vi "LJUD_eTCValuesB.vi"(5 "aResetCounters":bool[](array[boolean]), 6 "aTimerValues Write":dbl[](array[numeric]) format="%.2f", 7 "aReadCounters":bool[](array[boolean]), 8 "error in":errorcluster, 9 "aUpdateResetTimers":bool[](array[boolean]), 10 "aReadTimers":bool[](array[boolean]), 11 "Handle In":i32) -> (0 "error out":errorcluster, 1 "aCounterValues":dbl[](array[numeric]) format="%.2f", 2 "aTimerValues Read":dbl[](array[numeric]) format="%.2f", 3 "Handle Out":i32)   [LabVIEW 2021]
doc: "This version of eTCValues uses booleans\nfor some parameters.\n\nThis is an e-function that can update\nand read all the timers and counters\nin a single call. A somewhat complex\nfunction, but can help reinforce the\ninteraction between the different timers\nand counters on the device.\n\nSee Sections 4.2 and 4.3 of the device's\ndatasheet for more information."
uses:
  labjackud.dll
panel:
  # "This version of eTCValues uses booleans\nfor some parameters.  This makes for\nmore readable programs."
  # "This version of eTCValues uses booleans\nfor some parameters.\n\nThis is an e-function that can update\nand read all the timers and counters\nin a single call.  A somewhat complex\nfunction, but can help reinforce the\ninteraction between the different timers\nand counters on the device.\n\nSee Sections 4.2 and 4.3 of the device's\ndatasheet for more information."
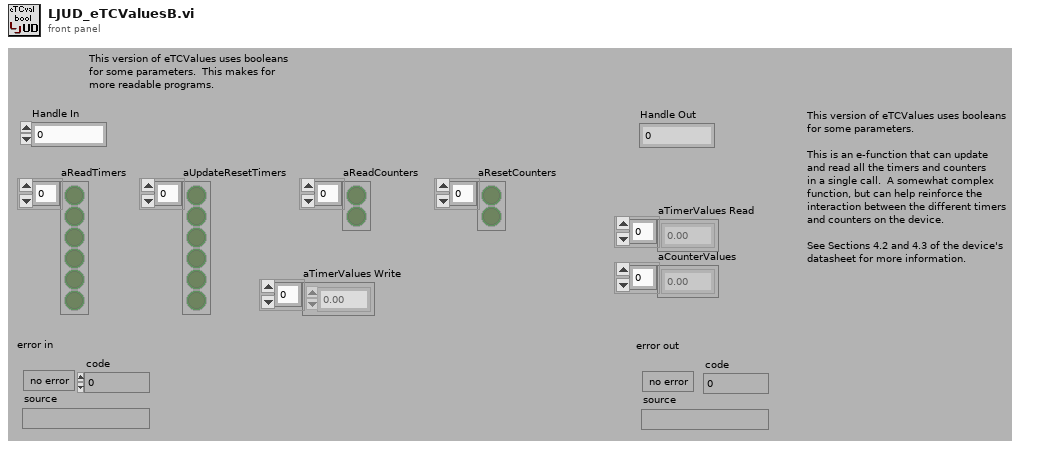
[diagram p1: front panel]
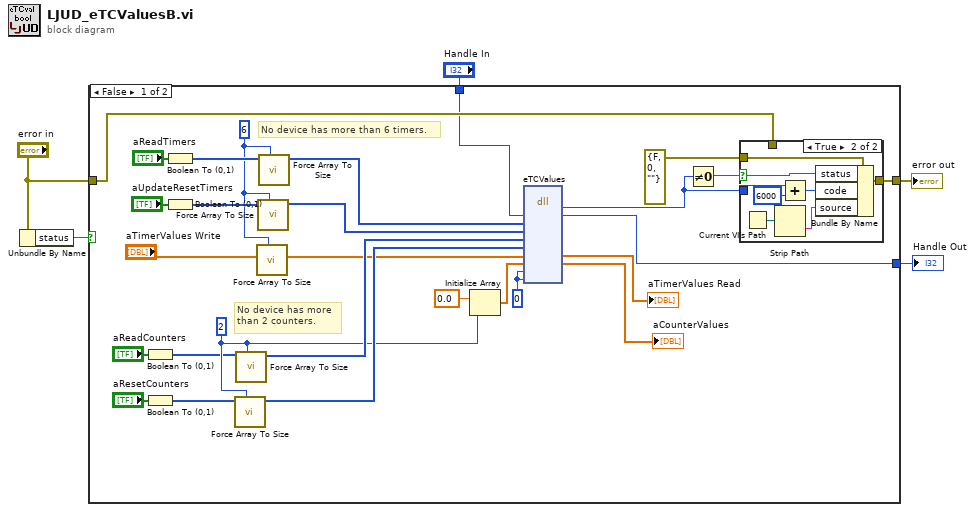
[diagram p0: block diagram]
diagram:
  n1 = Unbundle By Name("error in") -> ("status"=w4:bool)
  n2 = case shown="False" w4 {
    tunnel: [w30 w44] -> w5
    tunnel: "error in" -> [w29 w44]
    tunnel: "Handle In" -> [w7 w43]
    tunnel: [w6 w43] -> w1
    frame False {
      w9 = 6 ("# Elements")
      w23 = 2 ("# Elements")
      w26 = 0 ("GoError")
      # "No device has more\nthan 2 counters."
      # "No device has more than 6 timers."
      n3 = Boolean To (0,1)(Boolean="aReadCounters") -> (0, 1=w14:i16[])
      n4 = Boolean To (0,1)(Boolean="aResetCounters") -> (0, 1=w12:i16[])
      n5 = Boolean To (0,1)(Boolean="aReadTimers") -> (0, 1=w16:i16[])
      n6 = Boolean To (0,1)(Boolean="aUpdateResetTimers") -> (0, 1=w15:i16[])
      n7 = call "Force Array To Size.vi"("# Elements"=w23, "I32 Array In"=w12) -> ("I32 Array Out"=w24:i32[])  [unwired: 6 in, 3 out]
      n8 = call "Force Array To Size.vi"("# Elements"=w23, "I32 Array In"=w14) -> ("I32 Array Out"=w25:i32[])  [unwired: 6 in, 3 out]
      n9 = call "Force Array To Size.vi"("# Elements"=w9, "DBL Array In"="aTimerValues Write") -> ("DBL Array Out"=w8:dbl[])  [unwired: 6 in, 3 out]
      n10 = call "Force Array To Size.vi"("# Elements"=w9, "I32 Array In"=w15) -> ("I32 Array Out"=w20:i32[])  [unwired: 6 in, 3 out]
      n11 = call "Force Array To Size.vi"("# Elements"=w9, "I32 Array In"=w16) -> ("I32 Array Out"=w21:i32[])  [unwired: 6 in, 3 out]
      n12 = Initialize Array(0.0 ("Element Data"), w23) -> (w22:dbl[])
      n13 = dll-call lib="labjackud.dll" fn="eTCValues"("Handle"=w7, "aReadTimers"=w21, "aUpdateResetTimers"=w20, "aReadCounters"=w25, "aResetCounters"=w24, "aTimerValues"=w8, "aCounterValues"=w22, "Reserved1"=w26, "Reserved2"=w26) -> (w31:i32, "Handle"=w6:i32, "aTimerValues"=→"aTimerValues Read":dbl[], "aCounterValues"=→"aCounterValues":dbl[])  [unwired: 9 in, 2 out]
      n14 = Not Equal To 0?(x=w31) -> (x != 0?=w32:bool)
      n15 = case shown="True" w32 {
        selector: w32 -> [_ w41]
        tunnel: [w34 w42] -> w30
        tunnel: errorcluster {"status"=FALSE, "code"=0, "source"=""} ("error IO") -> [_ w40]
        tunnel: w31 -> [_ w36]
        tunnel: w29 -> [w34 _]
        frame False {
        }
        frame True {
          n16 = Current VI's Path() -> (path=w38:path)
          n17 = Strip Path(path=w38) -> (name=w39:string)  [unwired: 1 out]
          n18 = Add(x=w36, y=6000) -> (x+y=w37:i32)
          n19 = Bundle By Name(cluster=w40, "status"=w41, "code"=w37, "source"=w39) -> (w42:errorcluster)
        }
      }
    }
    frame True {
    }
  }
  "error out" <- w5
  "Handle Out" <- w1
